vi "Tool Q LEIN High G try to q a retreive command.vi"(0 "LEIN custom reply Q":T1, 5 "Message index":i32, 9 "Axis":i32, 11 "error in (no error)":errorcluster) -> (14 "Tried to send":bool, 15 "error out":errorcluster)   [LabVIEW 2011]
uses:
  LEINmaster/Defenitions/LEIN custom reply Q.ctl
  LEINmaster/Defenitions/LEIN Reply Holder.ctl
  LEINmaster/Defenitions/LEIN CMD Cluster.ctl
  LEINmaster/Defenitions/LEIN CMD List.ctl
  LEINmaster/Defenitions/LEIN Structure variations.ctl
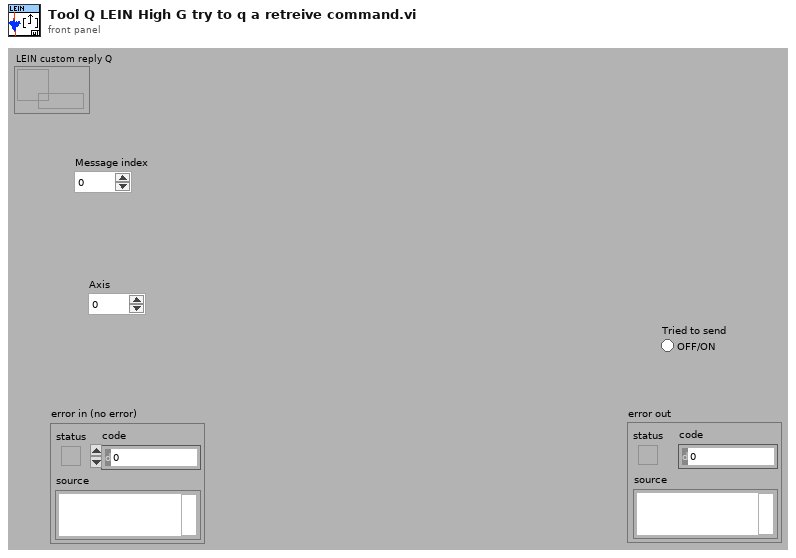
[diagram p1: front panel]
types:
  T1 = typedef "LEIN custom reply Q.ctl" = refnum<queue>
  T2 = enum16{"big-endian, network order", "native, host order", "little-endian"}
  T3 = typedef "LEIN Structure variations.ctl" = enum16{"LEIN08", "LEIN31", "LEIN63"}
  T4 = typedef "LEIN CMD Cluster.ctl" = cluster{"SID":u8, "ANF":bool, "CMD":T5, "DATA":u8[]}
  T5 = typedef "LEIN CMD List.ctl" = enum8{"ACTI", "TASK", "RES0", "STAT", "RES1", "RES2", "RES3", "USER"}
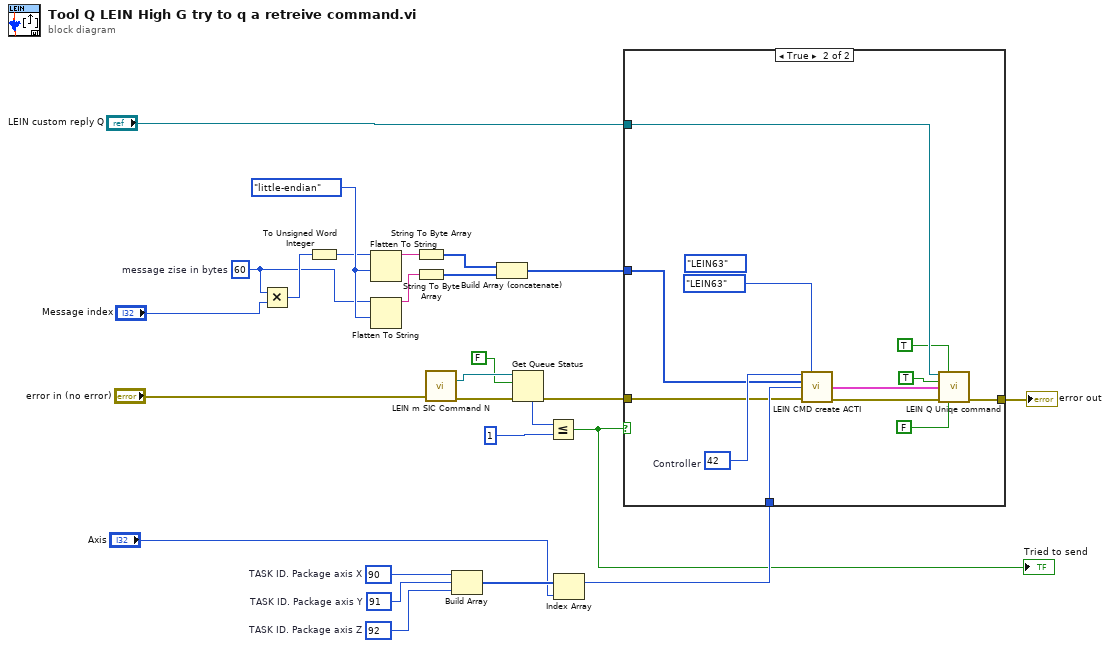
[diagram p0: block diagram]
diagram:
  w10 = u16 60  # message zise in bytes
  w16 = u8 92  # TASK ID. Package axis Z
  w17 = u8 91  # TASK ID. Package axis Y
  w21 = u8 90  # TASK ID. Package axis X
  w19 = T2."little-endian" ("byte order (0:big-endian, network order)")
  n1 = Multiply(x=w10, y="Message index") -> (x*y=w12:i32)
  n2 = To Unsigned Word Integer(number=w12) -> (unsigned 16bit integer=w11:u16)
  n3 = Flatten To String(anything=w11, byte order (0:big-endian, network order)=w19) -> (data string=w26:string)  [unwired: 2 in, 2 out]
  n4 = Flatten To String(anything=w10, byte order (0:big-endian, network order)=w19) -> (data string=w24:string)  [unwired: 2 in, 2 out]
  n5 = String To Byte Array(string=w26) -> (unsigned byte array=w25:u8[])
  n6 = String To Byte Array(string=w24) -> (unsigned byte array=w23:u8[])
  n7 = call "LEIN m SIC Command N.vi"("error in (no error)"="error in (no error)") -> ("queue out"=w9:refnum<queue>, "error out"=w6:errorcluster)  [unwired: 13 in]
  n8 = Build Array(w21, w17, w16) -> (w18:u8[])
  n9 = Build Array (concatenate)(w25, w23) -> (w20:u8[])
  n10 = Get Queue Status(queue=w9, return elements? (F)=FALSE, error in (no error)=w6) -> (error out=w7:errorcluster, # elements in queue=w4:i32)  [unwired: 6 out]
  n11 = Less Or Equal?(x=w4, y=1) -> (x <= y?=w2:bool)
  "Tried to send" <- w2
  n12 = Index Array(array=w18, index="Axis") -> (element=w15:u8)
  n13 = case shown="True" w2 {
    tunnel: [w27 w38] -> w22
    tunnel: w20 -> [_ w34]
    tunnel: w15 -> [_ w32]
    tunnel: w7 -> [w27 w31]
    tunnel: "LEIN custom reply Q" -> [_ w30]
    frame False {
    }
    frame True {
      w36 = u8 42  # Controller
      (unwired) LEIN_Structure_variations."LEIN63" ("LEIN Variation")
      n14 = call "LEIN CMD create ACTI.vi"("SID"=w36, "LEIN Variation"=LEIN_Structure_variations."LEIN63", "Data"=w34, "ACTI ID"=w32, "error in (no error)"=w31) -> ("CMD"=w33:T4, "error out"=w35:errorcluster)  [unwired: 9 in]
      n15 = call "LEIN Q Uniqe command.vi"("LEIN custom reply Q"=w30, "Retry on err (F)"=TRUE, "Custom Q(F)"=TRUE, "CMD"=w33, "error in"=w35, "priority(F)"=FALSE) -> ("error out"=w38:errorcluster)  [unwired: 9 in]
    }
  }
  "error out" <- w22
